vi "move axes.vi"(8 "error in":errorcluster, 10 "stage to move":enum16{"both", "fine", "coarse"}(ring), 11 "GPIB # (in): def. 6":string="6") -> (0 "error out":errorcluster, 3 "GPIB # (out)":string)   [LabVIEW 2017]
doc: "This tells the translation stage to go to the position that has previously been set."
uses:
  mc2mc4.llb/MC2/4  SendCommand.VI
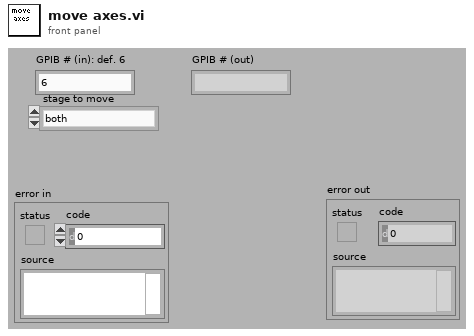
[diagram p1: front panel]
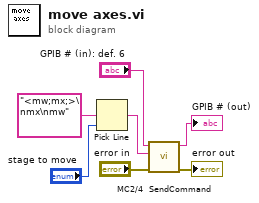
[diagram p0: block diagram]
diagram:
  n1 = Pick Line(multi-line string="<mw;mx;>\nmx\nmw", line index="stage to move") -> (output string=w4:string)  [unwired: 1 out]
  n2 = call "MC2/4  SendCommand.VI"("error in (no error)"="error in", "MC2 / MC4 Command"=w4, "GPIB # (in): def.6"="GPIB # (in): def. 6") -> ("error out"=→"error out":errorcluster, "GPIB # (out)"=→"GPIB # (out)":string)  [unwired: 7 out]
